vi "3 - get segment values from XY data.vi"() -> ()   [LabVIEW 2013]
uses:
  <vilib>/Utility/file.llb/Read From Spreadsheet File (DBL).vi
  <vilib>/Utility/file.llb/Write To Spreadsheet File (I64).vi
panel:
  out "path":path
  out "size(s)":i32
  out "Numeric":i32
  out "file path (dialog if empty)":path
  in  "Array":path[](array[path])
  in  "XY and frame data":dbl[][](array[numeric])=array14019x5[70095 elements] format="%0.3f"
  in  "appended array 2":dbl[][](array[numeric])
  in  "speed":u32(slide)
  out "Image 3":T1(plugin-control)
  in  "AVI Path":path=path "E:/PhD work/PhD research work/Videos/Chen Jin vs Hu Yun (Edited).avi"
  in  "appended array":dbl[][](array[numeric])=array1939x5[9695 elements]
  in  "Frames XY (top/bottom)":dbl[][](array[numeric])
  out "Infered action indicators":string[][](array[string])
  out "Movement data from both players":i32[][](array[numeric])
  out "Top player court segment display 2":bool[][](array[boolean])
  out "count top":i32[](graph)
  out "count bottom":i32[](graph)
  out "trans top":i32[](graph)
  out "trans bottom":i32[](graph)
  in  "ON":bool
  out "Top player court segment display":bool[][](array[boolean])
  out "Top VIew":cluster{"Numeric":dbl, "Numeric":dbl}[](graph)
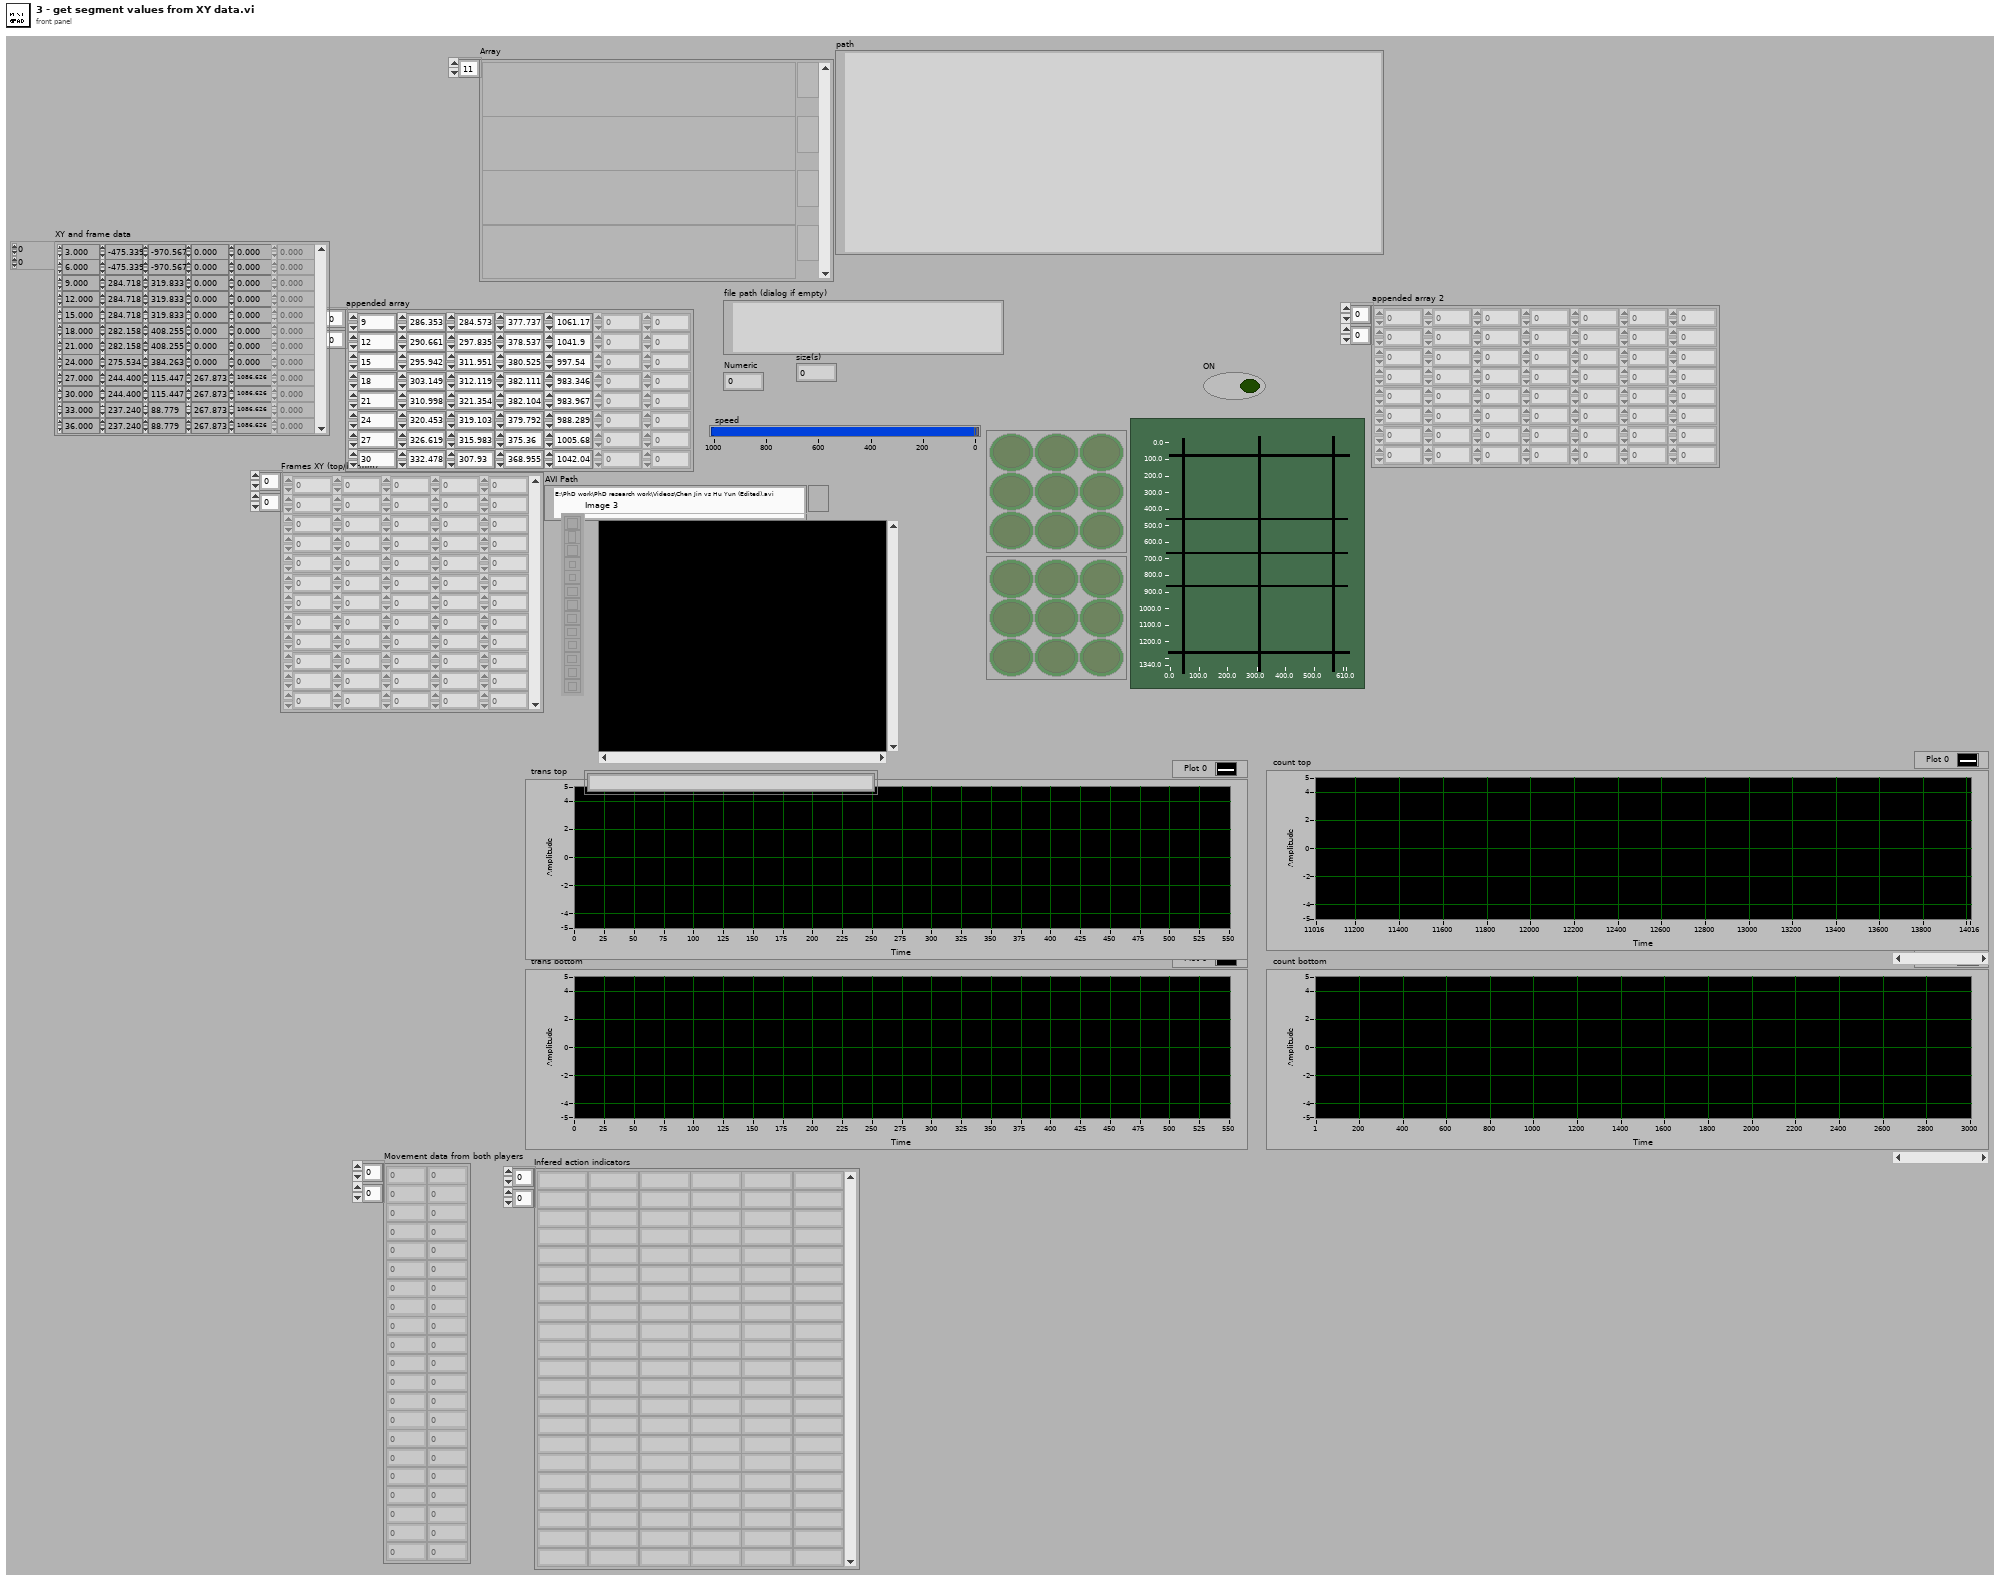
[diagram p1: front panel]
types:
  T1 = typedef "IMAQ Image.ctl" = refnum<image>
  T2 = typedef "Image Type" = u32
  T3 = typedef "AviRefnum.ctl" = refnum<k1>
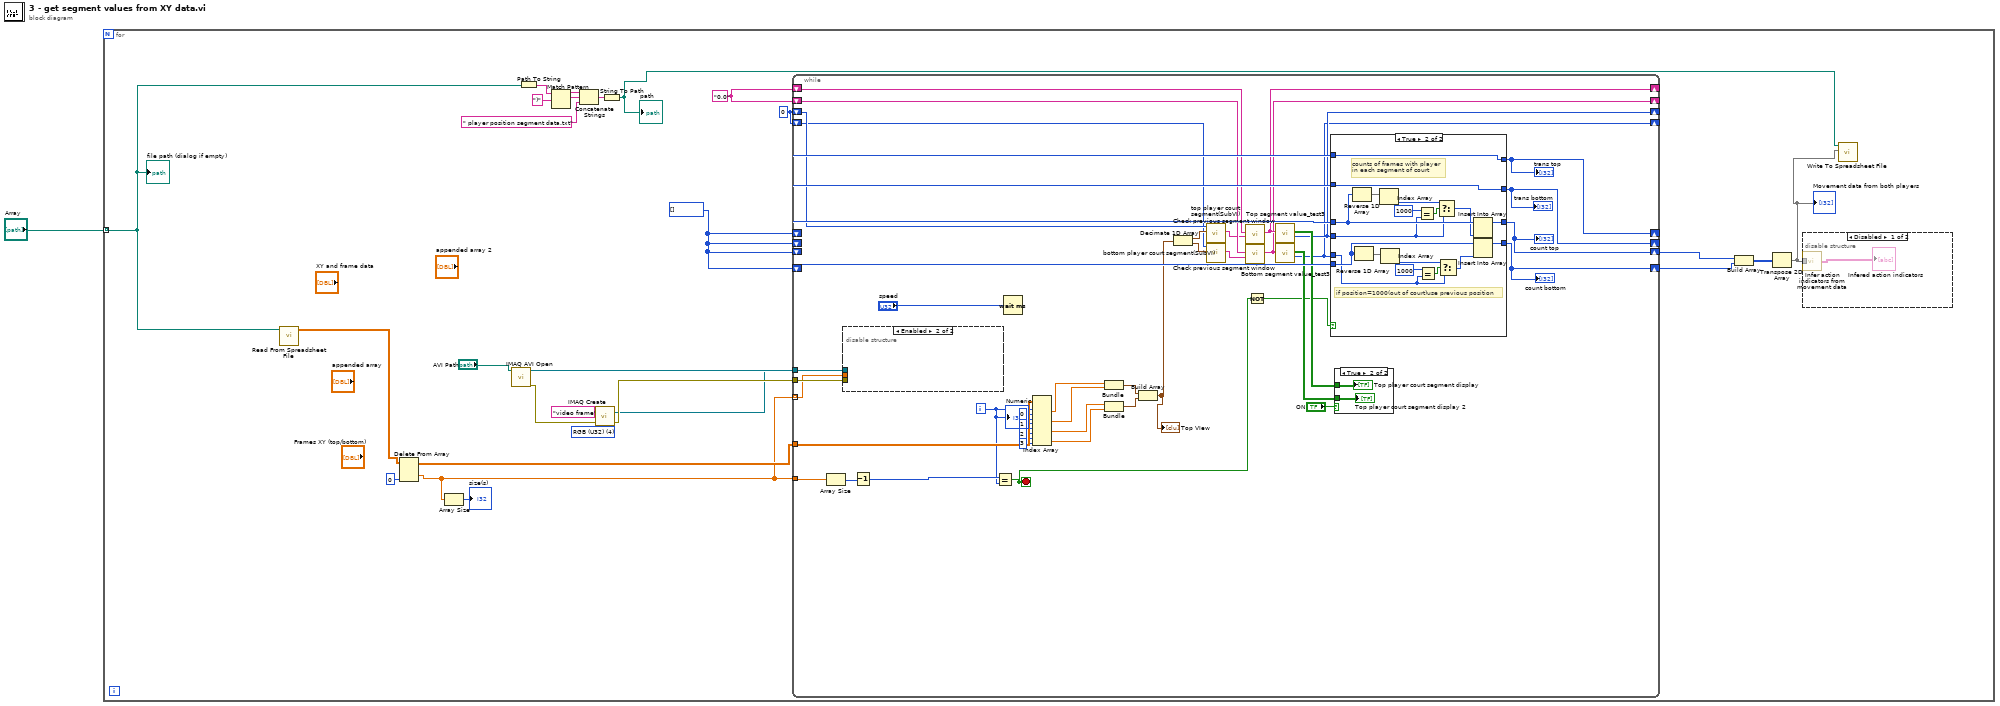
[diagram p0: block diagram]
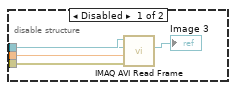
[diagram p3: hidden frame]
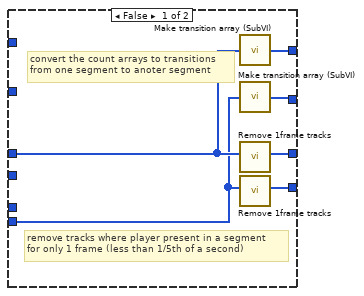
[diagram p4: hidden frame]
diagram:
  n1 = for {
    tunnel: "Array" -> [w7] mode=indexing
    w14 = 0 ("Top player segment value")
    w19 = T2 4 items=["Grayscale (U8)", "Grayscale (I16)", "Grayscale (SGL)", "Complex (CSG)", "RGB (U32)", "HSL (U32)", "RGB (U64)", "Grayscale (U16)"] ("Image Type")
    w28 = "0,0" ("Player segment position")
    w27 = i32[] [] ("input array")
    n2 = call-poly <vilib>:"Read From Spreadsheet File.vi"("file path (dialog if empty)"=w7) -> ("all rows"=w6:dbl[][])  [unwired: 6 in, 4 out]
    n3 = Delete From Array(array=w6, index (col)=0 ("disabled index (col)")) -> (deleted portion=w4:dbl[], array with subset deleted=w22:dbl[][])  [unwired: 2 in]
    n4 = Array Size(array=w4) -> (size(s)=→"size(s)":i32)
    n5 = call "IMAQ AVI Open"("AVI Path"="AVI Path") -> ("error out"=w17:errorcluster, "Avi Refnum"=w20:T3)  [unwired: 9 in]
    n6 = Path To String(path=w7) -> (string=w9:string)
    n7 = Match Pattern(string=w9, regular expression=")") -> (before substring=w11:string, match substring=w12:string)  [unwired: 1 in, 2 out]
    n8 = Concatenate Strings(w11, w12, " player position segment data.txt" ("regular expression")) -> (w13:string)
    n9 = call "IMAQ Create"("Image Name"="video frame", "Image Type"=w19, "error in (no error)"=w17) -> ("New Image"=w15:T1, "error out"=w16:errorcluster)  [unwired: 2 in]
    n10 = String To Path(string=w13) -> (path=w5:path)
    "path" <- w5
    n11 = while {
      shift-right: [w56] -> w25
      shift-left: w27 -> [w71]
      shift-right: [w57] -> w24
      shift-left: w27 -> [w72]
      shift-right: [w63] -> _
      shift-left: w27 -> [w69]
      shift-right: [w68] -> _
      shift-left: w27 -> [w70]
      shift-right: [w59] -> _
      shift-left: w28 -> [w64]
      shift-right: [w60] -> _
      shift-left: w28 -> [w65]
      tunnel: w4 -> [w46]
      tunnel: w22 -> [w55]
      tunnel: w20 -> [w39]
      tunnel: w16 -> [w38]
      tunnel: w15 -> [w37]
      tunnel: w4 -> [w36] mode=indexing
      shift-right: [w34] -> _
      shift-left: w14 -> [w32]
      shift-right: [w33] -> _
      shift-left: w14 -> [w31]
      i -> [w43]
      stop <- w41 stop-if-true
      n12 = Array Size(array=w46) -> (size(s)=w45:i32)
      n13 = disable-structure shown="Enabled" {
        disable-tunnel: w39 -> [w81 _]
        disable-tunnel: w38 -> [w80 _]
        disable-tunnel: w37 -> [w79 _]
        disable-tunnel: w36 -> [w78 _]
        frame Disabled {
          n14 = call "IMAQ AVI Read Frame"("error in (no error)"=w80, "Frame Number"=w78, "Image"=w79, "Avi Refnum"=w81) -> ("Image Out"=→"Image 3":T1)  [unwired: 4 in, 3 out]
        }
        frame Enabled {
        }
      }
      n15 = Decrement(x=w45) -> (x-1=w44:i32)
      n16 = Equal?(x=w44, y=w43) -> (x = y?=w41:bool)
      n17 = Wait (ms)(milliseconds to wait="speed") -> ()  [unwired: 1 out]
      n18 = Index Array(array=w55, index (row) #1=w43, index (col) #1=0 ("disabled index (col)"), index (row) #2=w43, index (col) #2=1 ("disabled index (col)"), index (row) #3=w43, index (col) #3=2 ("disabled index (col)"), index (row) #4=w43, index (col) #4=3 ("disabled index (col)")) -> (element #1=w50:dbl, element #2=w49:dbl, element #3=w48:dbl, element #4=w47:dbl)
      n19 = Bundle(w50, w49) -> (w76:cluster{dbl, dbl})  [unwired: 1 in]
      n20 = Bundle(w48, w47) -> (w58:cluster{dbl, dbl})  [unwired: 1 in]
      n21 = Build Array(w76, w58) -> (w40:cluster{dbl, dbl}[])
      "Top VIew" <- w40
      n22 = Decimate 1D Array(w40) -> (w74:cluster{dbl, dbl}[], w75:cluster{dbl, dbl}[])
      n23 = call "top player court segment(SubVI).vi"("Top player position"=w74, "previous segment"=w32) -> ("Top player segment position"=w62:string)  [unwired: 9 in]
      n24 = call "bottom player court segment(SubVI).vi"("Bottom player position"=w75, "previous segment"=w31) -> ("Bottom player segment position"=w61:string)  [unwired: 9 in]
      n25 = call "Check previous segment window.vi"("Current player segment position"=w62, "Previous player segment position"=w65) -> ("Player segment position"=w60:string)  [unwired: 9 in]
      n26 = call "Check previous segment window.vi"("Current player segment position"=w61, "Previous player segment position"=w64) -> ("Player segment position"=w59:string)  [unwired: 9 in]
      n27 = Not(x=w41) -> (.not. x?=w42:bool)
      n28 = call "Top segment value_test3.vi"("Top player segment position"=w60) -> ("Top player segment value"=w34:i32, "Top player court segment display"=w67:bool[][])  [unwired: 9 in]
      n29 = call "Bottom segment value_test3.vi"("Bottom player segment position"=w59) -> ("Bottom player segment"=w33:i32, "Bottom player court segment display"=w66:bool[][])  [unwired: 9 in]
      n30 = case shown="True" w42 {
        tunnel: w72 -> [w85 w101]
        tunnel: w71 -> [w84 w91]
        tunnel: [w86 w102] -> w63
        tunnel: [w87 w103] -> w68
        tunnel: w33 -> [_ w88]
        tunnel: w34 -> [_ w96]
        tunnel: w70 -> [_ w103]
        tunnel: w69 -> [_ w102]
        tunnel: [w83 w105] -> w56
        tunnel: [w82 w104] -> w57
        frame False {
          # "convert the count arrays to transitions \nfrom one segment to anoter segment"
          # "remove tracks where player present in a segment \nfor only 1 frame (less than 1/5th of a second)"
          n31 = call "Make transition array (SubVI).vi"("count array in"=w85) -> ("Transition array out"=w86:i32[])
          n32 = call "Make transition array (SubVI).vi"("count array in"=w84) -> ("Transition array out"=w87:i32[])
          n33 = call "Remove 1frame tracks.vi"("count array in"=w85) -> ("count array out"=w82:i32[])  [unwired: 10 in]
          n34 = call "Remove 1frame tracks.vi"("count array in"=w84) -> ("count array out"=w83:i32[])  [unwired: 10 in]
        }
        frame True {
          # "if position=1000(out of court)use previous position"
          # "counts of frames with player\nin each segment of court"
          n35 = Reverse 1D Array(array=w101) -> (reversed array=w100:i32[])
          n36 = Reverse 1D Array(array=w91) -> (reversed array=w90:i32[])
          n37 = Index Array(array=w100) -> (element=w97:i32)  [unwired: 1 in]
          n38 = Index Array(array=w90) -> (element=w94:i32)  [unwired: 1 in]
          n39 = Equal?(x=1000 ("y"), y=w96) -> (x = y?=w98:bool)
          n40 = Equal?(x=1000 ("y"), y=w88) -> (x = y?=w93:bool)
          n41 = Select(t=w97, s=w98, f=w96) -> (s? t:f=w95:i32)
          n42 = Select(t=w94, s=w93, f=w88) -> (s? t:f=w89:i32)
          n43 = Insert Into Array(array=w101, new element=w95) -> (w104:i32[])  [unwired: 1 in]
          n44 = Insert Into Array(array=w91, new element=w89) -> (w105:i32[])  [unwired: 1 in]
        }
      }
      "trans bottom" <- w68
      "trans top" <- w63
      "count bottom" <- w56
      "count top" <- w57
      n45 = case shown="True" "ON" {
        tunnel: w67 -> [_ w107]
        tunnel: w66 -> [_ w106]
        frame False {
        }
        frame True {
          "Top player court segment display" <- w107
          "Top player court segment display 2" <- w106
        }
      }
      "Numeric" <- w43
    }
    n46 = Build Array(w24, w25) -> (w26:i32[][])
    n47 = Transpose 2D Array(2D array=w26) -> (transposed array=w2:i32[][])
    "Movement data from both players" <- w2
    n48 = disable-structure shown="Disabled" {
      disable-tunnel: w2 -> [w29 _]
      frame Disabled {
        n49 = call "Infer action indicators from movement data.vi"("movement data from both players"=w29) -> ("Infered action indicators"=→"Infered action indicators":string[][])
      }
      frame Enabled {
      }
    }
    n50 = call-poly <vilib>:"Write To Spreadsheet File.vi"("2D data"=w2, "file path (dialog if empty)"=w5) -> ()  [unwired: 6 in, 1 out]
    "file path (dialog if empty)" <- w7
  }
